vi "Data.Engine.Write Data to HW.vi"(8 "error in":errorcluster, 11 "Plugin Data Access in":refnum<class "Plugin Data Access.lvclass">) -> (0 "error out":errorcluster, 3 "Plugin Data Access out":refnum<class "Plugin Data Access.lvclass">)   [LabVIEW 2024, in "VS Plugin Inline Async API.lvlib" / "Plugin Data Access.lvclass"]
uses:
  Plugin Data Access.lvclass
  Plugin Data Access.lvclass/Plugin Data Access.ctl
  Read/Read.lvclass
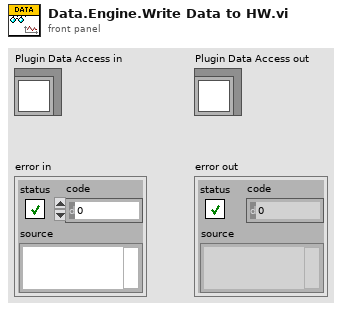
[diagram p1: front panel]
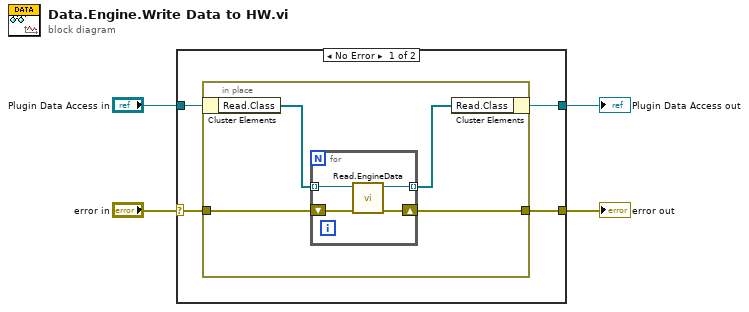
[diagram p0: block diagram]
diagram:
  n1 = case shown="No Error" "error in" {
    selector: "error in" -> [w7 w18]
    tunnel: [w8 w18] -> w3
    tunnel: [w6 w17] -> w1
    tunnel: "Plugin Data Access in" -> [w5 w17]
    frame No Error {
      n2 = in-place {
        in-place-border: w7 -> [w11]
        in-place-border: [w12] -> w8
        n3 = in-place-cluster #1(w5) -> ("Read.Class"=w10:refnum<class "Read.lvclass">[])
        n4 = for {
          tunnel: w10 -> [w14] mode=indexing
          shift-right: [w15] -> w12
          shift-left: w11 -> [w16]
          tunnel: [w13] -> w9 mode=indexing
          n5 = call "Read.EngineData.vi"("error in"=w16, "Read in"=w14) -> ("error out"=w15:errorcluster, "Read out"=w13:refnum<class "Read.lvclass">)  [unwired: 8 in]
        }
        n6 = in-place-cluster #1("Read.Class"=w9) -> (w6:refnum<class "Plugin Data Access.lvclass">)
      }
    }
    frame Error {
    }
  }
  "error out" <- w3
  "Plugin Data Access out" <- w1
